vi "Lab 1 Read Oscilloscope.vi"() -> ()   [LabVIEW 2015]
uses:
  <instrlib>/Siglent SDS 1000 2000 Series/Public/Data/Read Waveform Measurement (Px)_corrected.vi
  <instrlib>/Siglent SDS 1000 2000 Series/Siglent SDS 1000 2000 Series.lvlib
panel:
  in  "Reset (True) 2":bool=TRUE
  in  "Reset (True)":bool=TRUE
  out "Meter":dbl(knob) scale=0.0..500.0
  out "Waveform Chart":dbl(graph)
  in  "Parameter (0: P1)":u16(ring) items=["P1", "P2", "P3", "P4", "P5"]
  in  "error in (no error)":errorcluster
  in  "VISA resource name":refnum<visa-resource-name>
  in  "stop":bool
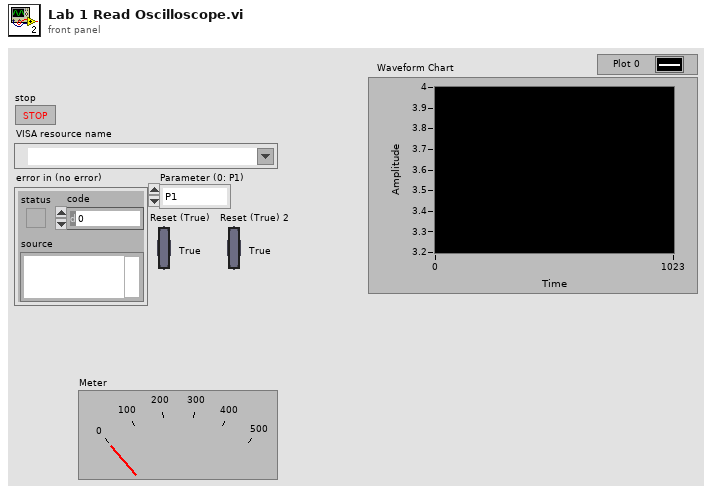
[diagram p1: front panel]
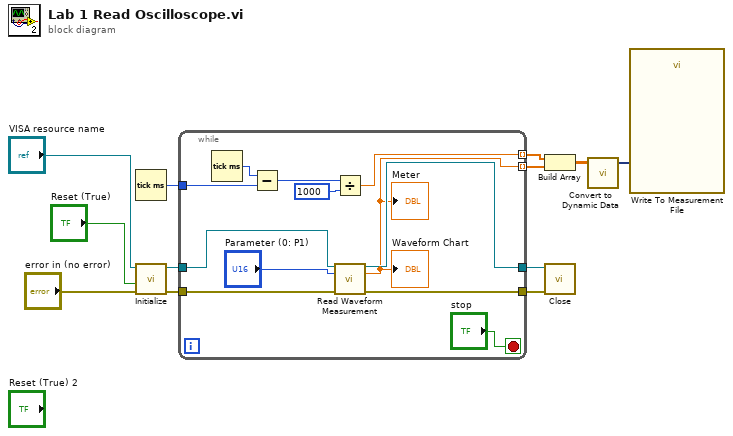
[diagram p0: block diagram]
diagram:
  n1 = Tick Count (ms)() -> (millisecond timer value=w8:u32)
  n2 = call <instrlib>:"Initialize.vi"("error in (no error)"="error in (no error)", "Reset (True)"="Reset (True)", "VISA resource name"="VISA resource name") -> ("error out"=w11:errorcluster, "VISA resource name out"=w2:refnum<visa-resource-name>)  [unwired: 7 in]
  n3 = while {
    tunnel: w11 -> [w23]
    tunnel: w2 -> [w22]
    tunnel: [w21] -> w1
    tunnel: [w20] -> w10
    tunnel: [w18] -> w5 mode=indexing
    tunnel: [w13] -> w6 mode=indexing
    tunnel: w8 -> [w17]
    stop <- "stop" stop-if-true
    n4 = Tick Count (ms)() -> (millisecond timer value=w16:u32)
    n5 = Subtract(x=w16, y=w17) -> (x-y=w15:u32)
    n6 = Divide(x=w15, y=1000) -> (x/y=w13:dbl)
    n7 = call-poly <instrlib>:"Read Waveform Measurement.vi"("VISA resource name"=w22, "Parameter (0: P1)"="Parameter (0: P1)", "error in (no error)"=w23) -> ("VISA resource name out"=w21:refnum<visa-resource-name>, "Value"=w18:dbl, "error out"=w20:errorcluster)  [unwired: 10 in]
    "Meter" <- w18
    "Waveform Chart" <- w18
  }
  n8 = Build Array(w6, w5) -> (w4:dbl[][])
  n9 = call <instrlib>:"Close.vi"("error in (no error)"=w10, "VISA resource name"=w1) -> ()  [unwired: 9 in, 1 out]
  n10 = call "Convert to Dynamic Data"("2D Array"=w4) -> ("Dynamic Data Type"=w3:dynamicdata)  [unwired: 3 in]
  n11 = call "Write To Measurement File"("Signals"=w3) -> ()  [unwired: 16 in, 3 out]
